vi "Set Column Headers.vi"(8 "error in (no error)":errorcluster, 10 "Column Header Strings[]":string[](array[string]), 11 "Tag Tree in":refnum<class "Tag Tree.lvclass">) -> (0 "error out":errorcluster, 3 "Tag Tree out":refnum<class "Tag Tree.lvclass">)   [LabVIEW 2020, in "Tree Helpers.lvlib" / "Tag Tree.lvclass"]
uses:
  Tag Tree.lvclass
  Tag Tree.lvclass/Tag Tree.ctl
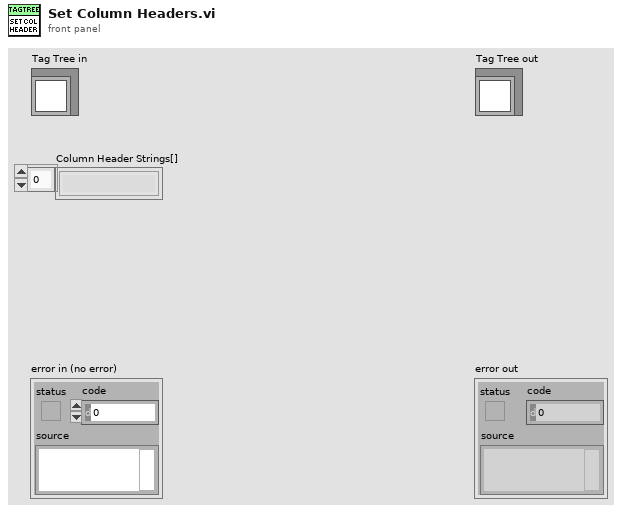
[diagram p1: front panel]
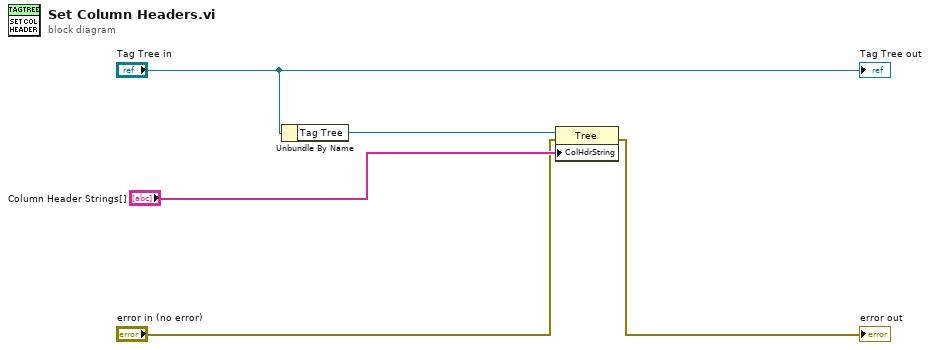
[diagram p0: block diagram]
diagram:
  n1 = Unbundle By Name("Tag Tree in") -> ("Tag Tree"=w4:refnum<vi>)
  n2 = property class="Tree"(reference=w4, error in="error in (no error)", "ColHdrString"="Column Header Strings[]") -> (error out=→"error out":errorcluster)  [unwired: 1 out]
  "Tag Tree out" <- "Tag Tree in"
